vi "Check ID for Message.vi"(7 "ID":string, 8 "error in (no error)":errorcluster, 11 "Minor Frame in":refnum<class "Minor Frame.lvclass">) -> (0 "error out":errorcluster, 2 "Msg Found?":bool, 3 "Minor Frame out":refnum<class "Minor Frame.lvclass">, 5 "Message":refnum<class "Message.lvclass">)   [LabVIEW 2020, in "BCI-1553 API.lvlib" / "Minor Frame.lvclass"]
doc: "Checks if the supplied ID is present in the list of messages.\nIf the message is found, it will be returned to the caller."
uses:
  Minor Frame.lvclass
  Message/Message.lvclass
  Minor Frame.lvclass/Minor Frame.ctl
  Dependencies/Registry/Registry.lvclass/Registry.ctl
  Dependencies/Registry/Registry.lvclass
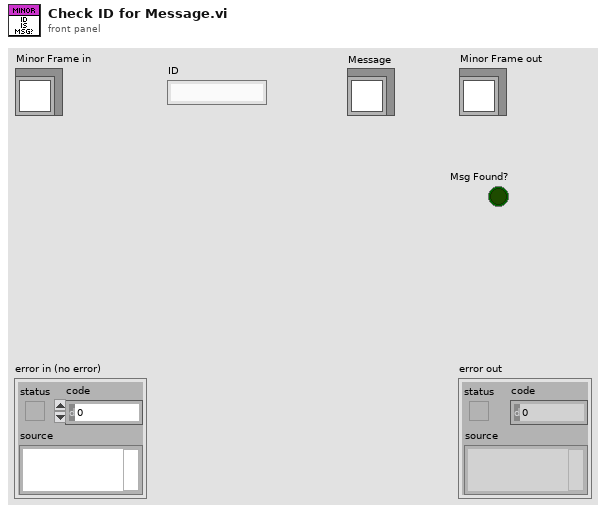
[diagram p1: front panel]
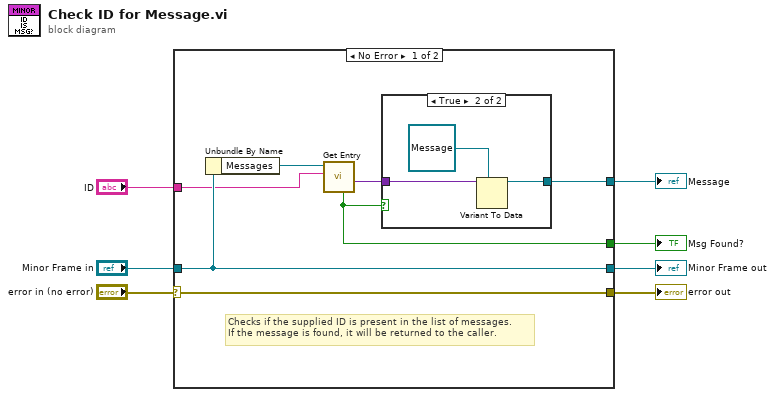
[diagram p0: block diagram]
diagram:
  n1 = case shown="No Error" "error in (no error)" {
    selector: "error in (no error)" -> [w14 w19]
    tunnel: [w14 w19] -> w4
    tunnel: [w13 w18] -> w5
    tunnel: "Minor Frame in" -> [w13 w18]
    tunnel: "ID" -> [w11 _]
    tunnel: [w9 _] -> w1
    tunnel: [w8 _] -> w2
    frame No Error {
      # "Checks if the supplied ID is present in the list of messages.\nIf the message is found, it will be returned to the caller."
      n2 = Unbundle By Name(w13) -> ("Messages"=w12:refnum<class "Registry.lvclass">)
      n3 = call "Get Entry.vi"("Key"=w11, "Registry in"=w12) -> ("Value"=w10:variant, "Found?"=w9:bool)  [unwired: 6 in, 2 out]
      n4 = case shown="True" w9 {
        tunnel: w10 -> [_ w17]
        tunnel: [_ w15] -> w8
        frame False {
        }
        frame True {
          n5 = Variant To Data(type=refnum<class "Message.lvclass"> refnum ("Message"), Variant=w17) -> (data=w15:refnum<class "Message.lvclass">)  [unwired: 1 in, 1 out]
        }
      }
    }
    frame Error {
    }
  }
  "error out" <- w4
  "Minor Frame out" <- w5
  "Message" <- w2
  "Msg Found?" <- w1
